vi "Poly_fit.vi"(0 "Input Y array":dbl[](array[numeric]) format="%.4f", 2 "Input X array":dbl[](array[numeric]) format="%.3f", 4 "polynomial order":i32=2, 5 "Point selector":cluster{"Y":dbl, "X":dbl, "switch":bool}[](array[cluster]) {"X" format="%.2f"; "Y" format="%.2f"}) -> (1 "Coefficients":dbl[](array[numeric]) format="%.2f", 6 "Calib const":string[][](array[string]), 7 "Calibration plot":cluster{cluster{dbl, dbl}[]}[](graph), 8 "Point selector":cluster{"Y":dbl, "X":dbl, "switch":bool}[](array[cluster]) {"X" format="%.2f"; "Y" format="%.2f"})   [LabVIEW 2010]
uses:
  <vilib>/Analysis/NI_AALPro.lvlib
  <vilib>/Analysis/NI_AALBase.lvlib
panel:
  in  "Type":cluster{"Y":dbl, "X":dbl, "switch":bool}={"Y"=10.144154930121, "X"=9.20412, "switch"=FALSE} {"X" format="%.2f"; "Y" format="%.2f"}
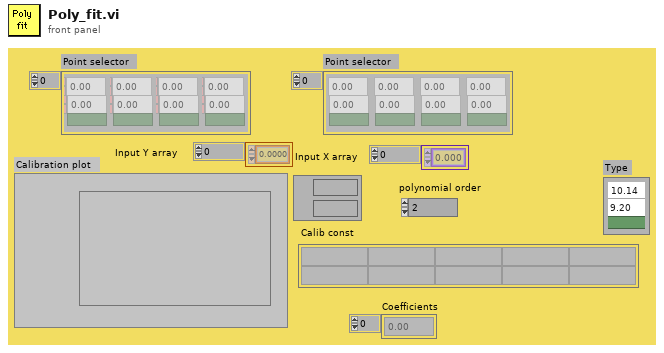
[diagram p1: front panel]
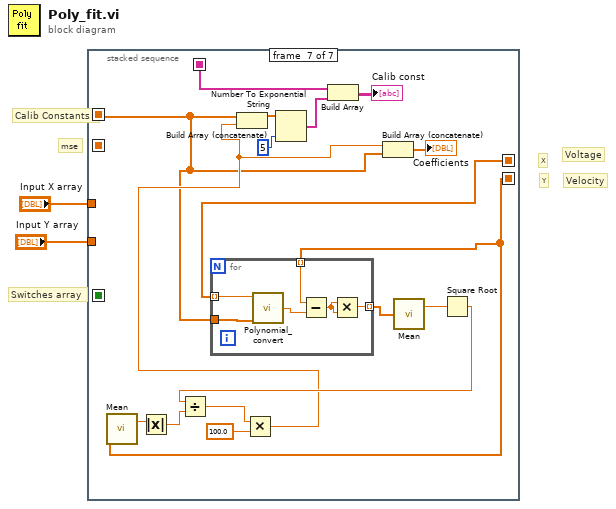
[diagram p0: block diagram]
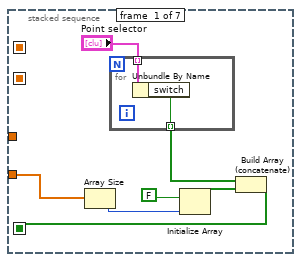
[diagram p2: hidden frame]
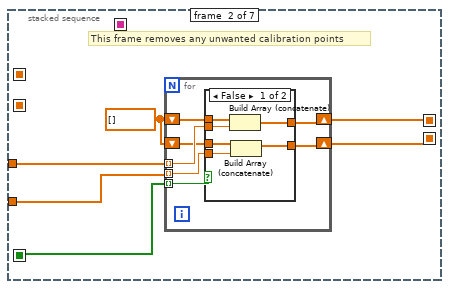
[diagram p3: hidden frame]
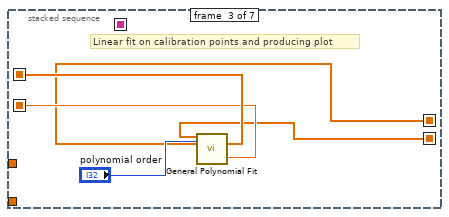
[diagram p5: hidden frame]
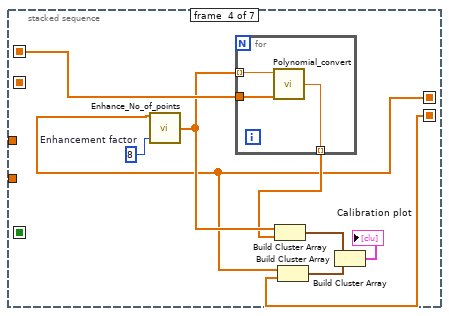
[diagram p6: hidden frame]
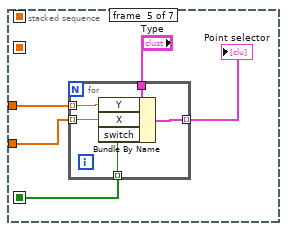
[diagram p7: hidden frame]
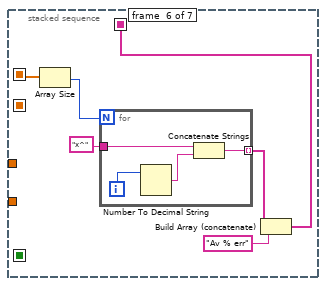
[diagram p8: hidden frame]
diagram:
  # "mse"
  # "Calib Constants"
  # "Voltage"
  # "Velocity"
  # "Switches array"
  # "X"
  # "Y"
  n1 = stacked-sequence {
    seq-local: [_ w17 _ _ _ _ _] -> [_ _ w34 w39 _ _ w71]
    seq-local: [_ w16 _ _ _ _ _] -> [_ _ w33 w38 _ _ w73]
    seq-local: [w7 _ _ _ _ _ _] -> [_ w13 _ _ w51 _ _]
    seq-local: [_ _ w37 _ _ _ _] -> [_ _ _ w42 _ w63 w70]
    seq-local: [_ _ w36 _ _ _ _] -> [_ _ _ _ _ _ _]
    seq-local: [_ _ _ _ _ w60 _] -> [_ _ _ _ _ _ w83]
    tunnel: "Input Y array" -> [w3 w14 _ _ w52 _ _]
    tunnel: "Input X array" -> [_ w15 _ _ w53 _ _]
    frame #0 {
      n2 = Array Size(array=w3) -> (size(s)=w5:i32)
      n3 = for {
        tunnel: "Point selector" -> [w11] mode=indexing
        tunnel: [w10] -> w8 mode=indexing
        n4 = Unbundle By Name(w11) -> ("switch"=w10:bool)
      }
      n5 = Initialize Array(FALSE, w5) -> (w4:bool[])
      n6 = Build Array (concatenate)(w8, w4) -> (w7:bool[])
    }
    frame #1 {
      w12 = dbl[] []
      # "This frame removes any unwanted calibration points"
      n7 = for {
        shift-right: [w18] -> w16
        shift-left: w12 -> [w20]
        shift-right: [w19] -> w17
        shift-left: w12 -> [w21]
        tunnel: w13 -> [w22] mode=indexing
        tunnel: w14 -> [w23] mode=indexing
        tunnel: w15 -> [w24] mode=indexing
        n8 = case shown="False" w22 {
          tunnel: [w25 w31] -> w18
          tunnel: [w26 w32] -> w19
          tunnel: w20 -> [w27 w31]
          tunnel: w21 -> [w28 w32]
          tunnel: w23 -> [w29 _]
          tunnel: w24 -> [w30 _]
          frame False {
            n9 = Build Array (concatenate)(w28, w30) -> (w26:dbl[])
            n10 = Build Array (concatenate)(w27, w29) -> (w25:dbl[])
          }
          frame True {
          }
        }
      }
    }
    frame #2 {
      # "Linear fit on calibration points and producing plot"
      n11 = call <vilib>:"General Polynomial Fit.vi"("Y"=w33, "polynomial order"="polynomial order", "X"=w34) -> ("Polynomial Coefficients"=w37:dbl[], "residue"=w36:dbl)  [unwired: 9 in, 2 out]
    }
    frame #3 {
      w43 = 8  # Enhancement factor
      n12 = call "Enhance_No_of_points.vi"("Enhancement factor"=w43, "Input"=w39) -> ("Output"=w41:dbl[])  [unwired: 3 out]
      n13 = for {
        tunnel: w42 -> [w49]
        tunnel: w41 -> [w48] mode=indexing
        tunnel: [w47] -> w40 mode=indexing
        n14 = call "Polynomial_convert.vi"("Calib constants"=w49, "Voltage"=w48) -> ("Eng Values"=w47:dbl)  [unwired: 4 out]
      }
      n15 = Build Cluster Array(w41, w40) -> (w46:cluster{dbl, "Eng Values":dbl}[])
      n16 = Build Cluster Array(w39, w38) -> (w45:cluster{dbl, dbl}[])
      n17 = Build Cluster Array(w46, w45) -> (→"Calibration plot":cluster{cluster{dbl, "Eng Values":dbl}[]}[])
    }
    frame #4 {
      n18 = for {
        tunnel: "Type" -> [w59]
        tunnel: w53 -> [w58] mode=indexing
        tunnel: w52 -> [w57] mode=indexing
        tunnel: w51 -> [w56] mode=indexing
        tunnel: [w55] -> w50 mode=indexing
        n19 = Bundle By Name(cluster=w59, "Y"=w58, "X"=w57, "switch"=w56) -> (w55:cluster{"Y":dbl, "X":dbl, "switch":bool})
      }
      "Point selector" <- w50
    }
    frame #5 {
      n20 = Array Size(array=w63) -> (size(s)=w62:i32)
      n21 = for {
        N: w62 -> [_]
        tunnel: "x^" -> [w67]
        tunnel: [w66] -> w61 mode=indexing
        i -> [w69]
        n22 = Number To Decimal String(number=w69) -> (decimal integer string=w68:string)  [unwired: 1 out]
        n23 = Concatenate Strings(w67, w68) -> (w66:string)
      }
      n24 = Build Array (concatenate)(w61, "Av % err") -> (w60:string[])
    }
    frame #6 {
      n25 = call <vilib>:"Mean.vi"("X"=w73) -> ("mean"=w80:dbl)  [unwired: 1 out]
      n26 = Absolute Value(x=w80) -> (abs(x)=w77:dbl)
      n27 = for {
        tunnel: w70 -> [w92]
        tunnel: w71 -> [w91] mode=indexing
        tunnel: w73 -> [w89] mode=indexing
        tunnel: [w87] -> w75 mode=indexing
        n28 = call "Polynomial_convert.vi"("Calib constants"=w92, "Voltage"=w91) -> ("Eng Values"=w90:dbl)  [unwired: 4 out]
        n29 = Subtract(x=w89, y=w90) -> (x-y=w88:dbl)
        n30 = Multiply(x=w88, y=w88) -> (x*y=w87:dbl)
      }
      n31 = call <vilib>:"Mean.vi"("X"=w75) -> ("mean"=w74:dbl)  [unwired: 1 out]
      n32 = Square Root(x=w74) -> (sqrt(x)=w78:dbl)
      n33 = Divide(x=w78, y=w77) -> (x/y=w76:dbl)
      n34 = Multiply(x=w76, y=100.0) -> (x*y=w72:dbl)
      n35 = Build Array (concatenate)(w70, w72) -> (w86:dbl[])
      n36 = Number To Exponential String(number=w86, precision (6)=i16 5) -> (E-format string=w85:string[])  [unwired: 2 out]
      n37 = Build Array(w83, w85) -> (→"Calib const":string[][])
      n38 = Build Array (concatenate)(w72, w70) -> (→"Coefficients":dbl[])
    }
  }
